vi "Equi-Ripple LowPass (DBL).vi"(0 "# of taps":i32=32, 1 "pass freq":dbl=0.2 format="%0.2f", 2 "stop freq":dbl=0.25 format="%0.2f", 3 "sampling freq: fs":dbl=1.0 format="%0.2f", 5 "X":dbl[](array[numeric])) -> (4 "error":i32, 7 "Filtered X":dbl[](array[numeric]))   [LabVIEW 2014, in "NI_AALBase.lvlib"]
doc: "Generates a lowpass FIR filter with equi-ripple characteristics using the Parks-McClellan algorithm and the <B># of taps</B>, <B>pass freq</B>, <B>stop freq</B>, and <B>sampling freq: fs</B>. The Equi-Ripple LowPass VI then applies a linear-phase, lowpass filter to the input sequence <B>X</B> using the Convolution VI to obtain <B>Filtered X</B>. Wire data to the <B>X</B> input to determine the polymorphic instance to use or manually select the instance."
uses:
  NI_AALBase.lvlib
  1D Convolution (DBL).vi
  NI_AALPro.lvlib
panel:
  # "Equi-Ripple\n Lowpass FIR Filter"
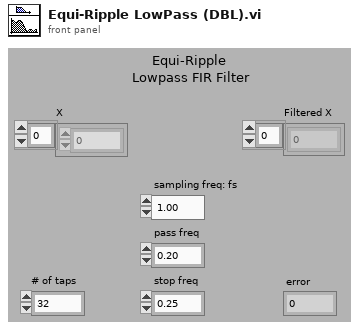
[diagram p1: front panel]
types:
  T1 = cluster{"Amplitude":dbl, "DC":dbl, "pass freq":dbl, "Weight":dbl}
  T2 = cluster{"Amplitude":dbl, "stop freq":dbl, dbl, "Weight":dbl}
  T3 = cluster{"Amplitude":dbl, "stop freq":dbl, "pass freq":dbl, "Weight":dbl}[]
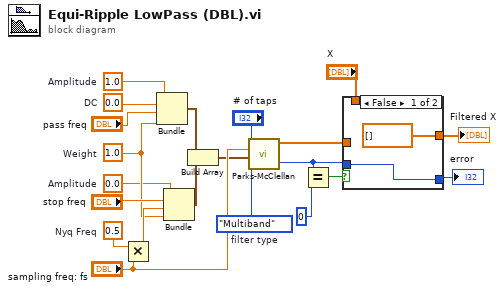
[diagram p0: block diagram]
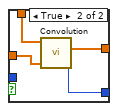
[diagram p2: hidden frame]
diagram:
  w1 = enum32{"Multiband", "Differentiator", "Hilbert"}."Multiband"  # filter type
  w18 = 0.5  # Nyq Freq
  w2 = 0.0  # Amplitude
  w3 = 1.0  # Weight
  w21 = 0.0  # DC
  w4 = 1.0  # Amplitude
  n1 = Multiply(x=w18, y="sampling freq: fs") -> (x*y=w17:dbl)
  n2 = Bundle("Amplitude"=w4, "DC"=w21, "pass freq"="pass freq", "Weight"=w3) -> (w16:T1)  [unwired: 1 in]
  n3 = Bundle("Amplitude"=w2, "stop freq"="stop freq", w17, "Weight"=w3) -> (w15:T2)  [unwired: 1 in]
  n4 = Build Array(w16, w15) -> (w8:T3)
  n5 = call "Parks-McClellan.vi"("filter type"=w1, "Band Parameters"=w8, "sampling freq: fs"="sampling freq: fs", "# of taps"="# of taps") -> ("error"=w5:i32, "h"=w7:dbl[])  [unwired: 1 out]
  n6 = Equal?(x=w5, y=0) -> (x = y?=w14:bool)
  n7 = case shown="False" w14 {
    tunnel: w5 -> [w23 _]
    tunnel: [w23 w24] -> w13
    tunnel: [dbl[] [] ("empty array") w25] -> w12
    tunnel: "X" -> [_ w27]
    tunnel: w7 -> [_ w26]
    frame False {
    }
    frame True {
      n8 = call-poly "Convolution.vi"("Y"=w26, "X"=w27) -> ("error"=w24:i32, "X * Y"=w25:dbl[])  [unwired: 8 in]
    }
  }
  "Filtered X" <- w12
  "error" <- w13
